vi "Get_XY_vectors_IMG.vi"(6 "TimeDelays,pixels":i32, 7 "Wavelength, pixels":i32, 8 "error in":errorcluster, 9 "ScalingYScalingFile":i64=1060864, 10 "ScalingXScalingFile":i64=1058816, 11 "path":path) -> (0 "error out":errorcluster, 2 "Y":dbl[](array[numeric]), 3 "X":dbl[](array[numeric]))   [LabVIEW 2015]
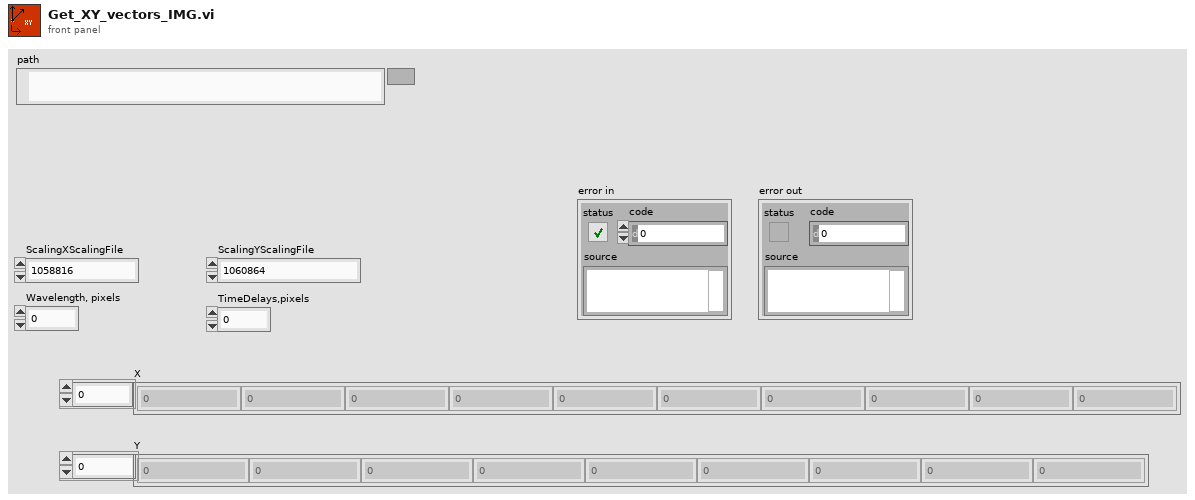
[diagram p1: front panel]
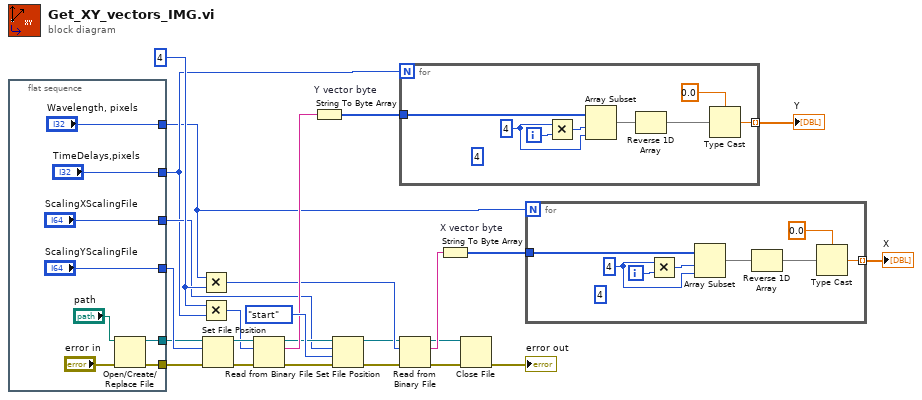
[diagram p0: block diagram]
diagram:
  w14 = 4 ("x")
  n1 = flat-sequence {
    tunnel: [w28] -> w12
    tunnel: [w27] -> w13
    tunnel: ["ScalingYScalingFile"] -> w17
    tunnel: ["ScalingXScalingFile"] -> w9
    tunnel: ["TimeDelays,pixels"] -> w5
    tunnel: ["Wavelength, pixels"] -> w1
    frame #0 {
      n2 = Open/Create/Replace File(file path (use dialog)="path", error in="error in") -> (refnum out=w28:refnum<file>, error out=w27:errorcluster)  [unwired: 4 in, 1 out]
    }
  }
  n3 = Multiply(x=w1, y=w14) -> (x*y=w15:i32)
  n4 = Multiply(x=w14, y=w5) -> (x*y=w16:i32)
  n5 = Set File Position(offset (in bytes) (0)=w17, refnum=w12, error in=w13) -> (refnum out=w22:refnum<file>, error out=w20:errorcluster)  [unwired: 1 in]
  n6 = Read from Binary File(8:w20, 10:w16, 11:w22) -> (0:w10:errorcluster, 2:w21:string, 3:w11:refnum<file>)  [unwired: 3 in, 1 out]
  n7 = String To Byte Array "Y vector byte"(string=w21) -> (unsigned byte array=w6:u8[])
  n8 = Set File Position(offset (in bytes) (0)=w9, refnum=w11, from (0:start)=enum16{"start", "end", "current"}."start" ("pos mode (0:2)"), error in=w10) -> (refnum out=w8:refnum<file>, error out=w7:errorcluster)
  n9 = for {
    N: w5 -> [_]
    tunnel: w6 -> [w41]
    tunnel: [w36] -> w4 mode=indexing
    i -> [w39]
    (unwired) 4 ("n")
    w37 = 4 ("x")
    n10 = Multiply(x=w37, y=w39) -> (x*y=w38:i32)
    n11 = Array Subset(array=w41, index=w38, length=w37) -> (w35:u8[])
    n12 = Reverse 1D Array(array=w35) -> (reversed array=w34:u8[])
    n13 = Type Cast(type=sgl 0.0, x=w34) -> (*(type *) &x=w36:sgl)
  }
  "Y" <- w4
  n14 = Read from Binary File(8:w7, 10:w15, 11:w8) -> (0:w19:errorcluster, 2:w24:string, 3:w23:refnum<file>)  [unwired: 3 in, 1 out]
  n15 = String To Byte Array "X vector byte"(string=w24) -> (unsigned byte array=w3:u8[])
  n16 = Close File(refnum=w23, error in=w19) -> (error out=→"error out":errorcluster)  [unwired: 1 out]
  n17 = for {
    N: w1 -> [_]
    tunnel: w3 -> [w49]
    tunnel: [w44] -> w2 mode=indexing
    i -> [w47]
    (unwired) 4 ("n")
    w45 = 4 ("x")
    n18 = Multiply(x=w45, y=w47) -> (x*y=w46:i32)
    n19 = Array Subset(array=w49, index=w46, length=w45) -> (w43:u8[])
    n20 = Reverse 1D Array(array=w43) -> (reversed array=w42:u8[])
    n21 = Type Cast(type=sgl 0.0, x=w42) -> (*(type *) &x=w44:sgl)
  }
  "X" <- w2
